vi "Transfer LSS Imaginary.vi"(1 "precision":u32, 2 "lambda":cdb[](array[numeric]) format="%.2f", 3 "beta":dbl[](array[numeric]) format="%.2f") -> (0 "formula linear combination":string)   [LabVIEW 2020, in "NI_Gmath.lvlib"]
uses:
  NI_Gmath.lvlib
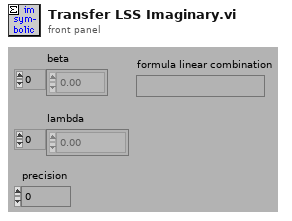
[diagram p1: front panel]
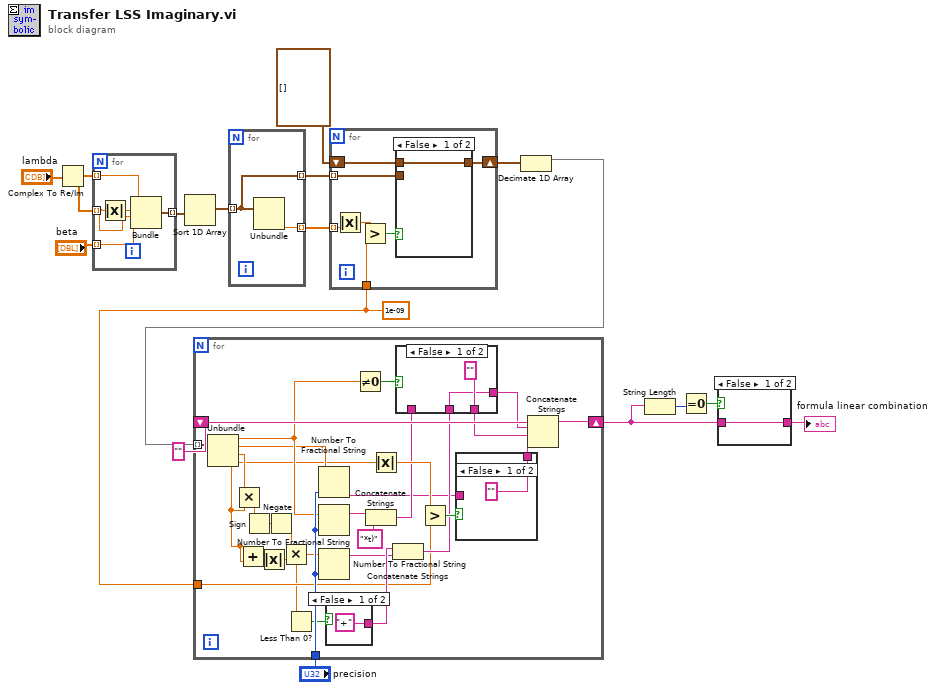
[diagram p0: block diagram]
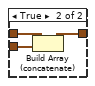
[diagram p2: hidden frame]
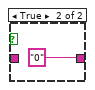
[diagram p3: hidden frame]
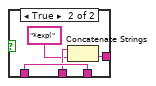
[diagram p4: hidden frame]
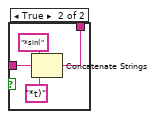
[diagram p5: hidden frame]
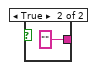
[diagram p6: hidden frame]
diagram:
  w2 = 1e-09
  n1 = Complex To Re/Im(x + iy="lambda") -> (x=w16:dbl[], y=w15:dbl[])
  n2 = for {
    tunnel: w16 -> [w23] mode=indexing
    tunnel: w15 -> [w19] mode=indexing
    tunnel: "beta" -> [w21] mode=indexing
    tunnel: [w20] -> w17 mode=indexing
    n3 = Absolute Value(x=w19) -> (abs(x)=w22:dbl)
    n4 = Bundle(w23, w22, w19, w21) -> (w20:cluster{dbl, dbl, dbl, dbl})  [unwired: 1 in]
  }
  n5 = Sort 1D Array(array=w17) -> (sorted array=w7:cluster{dbl, dbl, dbl, dbl}[])
  n6 = for {
    tunnel: w7 -> [w24] mode=indexing
    tunnel: [w25] -> w5 mode=indexing
    tunnel: [w24] -> w4 mode=indexing
    n7 = Unbundle(w24) -> (w25:dbl)  [unwired: 3 out]
  }
  n8 = for {
    shift-right: [w27] -> w3
    shift-left: cluster{dbl, dbl, dbl, dbl}[] [] -> [w28]
    tunnel: w5 -> [w32] mode=indexing
    tunnel: w2 -> [w30]
    tunnel: w4 -> [w26] mode=indexing
    n9 = Absolute Value(x=w32) -> (abs(x)=w31:dbl)
    n10 = Greater?(x=w31, y=w30) -> (0:w29:bool)
    n11 = case shown="False" w29 {
      tunnel: w28 -> [w33 w36]
      tunnel: [w33 w35] -> w27
      tunnel: w26 -> [_ w34]
      frame False {
      }
      frame True {
        n12 = Build Array (concatenate)(w36, w34) -> (w35:cluster{dbl, dbl, dbl, dbl}[])
      }
    }
  }
  n13 = Decimate 1D Array(w3) -> (w1:cluster{dbl, dbl, dbl, dbl}[])  [unwired: 1 out]
  n14 = for {
    shift-right: [w63] -> w12
    shift-left: "" -> [w64]
    tunnel: "precision" -> [w65]
    tunnel: w1 -> [w62] mode=indexing
    tunnel: w2 -> [w46]
    n15 = Unbundle(w62) -> (w47:dbl, w45:dbl, w44:dbl, w37:dbl)
    n16 = Multiply(x=w44, y=w37) -> (x*y=w43:dbl)
    n17 = Add(x=w37, y=w37) -> (x+y=w41:dbl)
    n18 = Sign(1:w43) -> (0:w42:dbl)
    n19 = Absolute Value(x=w41) -> (abs(x)=w39:dbl)
    n20 = Negate(x=w42) -> (-x=w38:dbl)
    n21 = Multiply(x=w38, y=w39) -> (x*y=w40:dbl)
    n22 = Less Than 0?(x=w40) -> (x < 0?=w53:bool)
    n23 = Number To Fractional String(number=w45, precision (6)=w65) -> (F-format string=w51:string)  [unwired: 2 in]
    n24 = Number To Fractional String(number=w47, precision (6)=w65) -> (F-format string=w49:string)  [unwired: 2 in]
    n25 = Number To Fractional String(number=w40, precision (6)=w65) -> (F-format string=w48:string)  [unwired: 2 in]
    n26 = case shown="False" w53 {
      tunnel: ["+" ""] -> w54
      frame False {
      }
      frame True {
      }
    }
    n27 = Not Equal To 0?(x=w47) -> (x != 0?=w55:bool)
    n28 = Concatenate Strings(w49, "*t)") -> (w59:string)
    n29 = Absolute Value(x=w37) -> (abs(x)=w60:dbl)
    n30 = Concatenate Strings(w54, w48) -> (w56:string)
    n31 = case shown="False" w55 {
      tunnel: w56 -> [w66 w70]
      tunnel: [w66 w68] -> w57
      tunnel: ["" w71] -> w58
      tunnel: w59 -> [_ w71]
      frame False {
      }
      frame True {
        n32 = Concatenate Strings(w70, "*exp(") -> (w68:string)
      }
    }
    n33 = Greater?(x=w60, y=w46) -> (0:w61:bool)
    n34 = case shown="False" w61 {
      tunnel: ["" w74] -> w52
      tunnel: w51 -> [_ w73]
      frame False {
      }
      frame True {
        n35 = Concatenate Strings("*sin(", w73, "*t)") -> (w74:string)
      }
    }
    n36 = Concatenate Strings(w64, w57, w58, w52) -> (w63:string)
  }
  n37 = String Length(string=w12) -> (length=w11:i32)
  n38 = Equal To 0?(x=w11) -> (x = 0?=w10:bool)
  n39 = case shown="False" w10 {
    tunnel: w12 -> [w79 _]
    tunnel: [w79 "0"] -> w9
    frame False {
    }
    frame True {
    }
  }
  "formula linear combination" <- w9
